vi "JTAG F-RAM Store Trims.vi"(8 "Control F-RAM Power?":bool=TRUE, 9 "Auto-Load this value?":bool=TRUE, 10 "Value to Store":u8 format="%02x", 11 "Trim Location":u16(ring) items=["PWR_TRIM_f0"=0, "PWR_TRIM_1"=1, "PWR_TRIM_2"=2, "PWR_TRIM_3"=3, "PWR_TRIM_4"=4, "PWR_TRIM_5"=5, "PWR_TRIM_6"=6, "PWR_TRIM_7"=7, "PWR_TRIM_8"=8, "PWR_TRIM_9"=9, "PWR_TRIM_10"=10, "STIM_BG_CTRL"=11, "STIM_CG_CTRL"=12, "STIM_PGO_CTRL"=13, "STIM_CM_CTRL"=14, "MICS_TX_RF_POWER"=20, "MICS_TXPORT_TXMODE"=21, "MICS_TXPORT_RXMODE"=22, "MICS_RXPORT_TXMODE"=23, "MICS_RXPORT_RXMODE"=24, "MICS_ANT_MATCH_1"=25, "MICS_ANT_MATCH_2"=26, "MICS_CHANNEL"=27, "MICS_TX_MODULATION"=28, "MICS_MAC_CALSELECT_1"=29, "MICS_MAC_CALSELECT_2"=30]) -> (0 "error out":errorcluster)   [LabVIEW 2009]
panel:
  # "Yes"
  # "No"
  # "Yes"
  # "No"
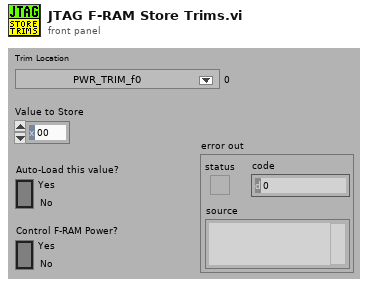
[diagram p1: front panel]
types:
  T1 = enum16{"Power UP", "Power DN", "Read Single", "Write Single", "Read Block", "Write Block", "Read SR", "Write SR", "Send Opcode"}
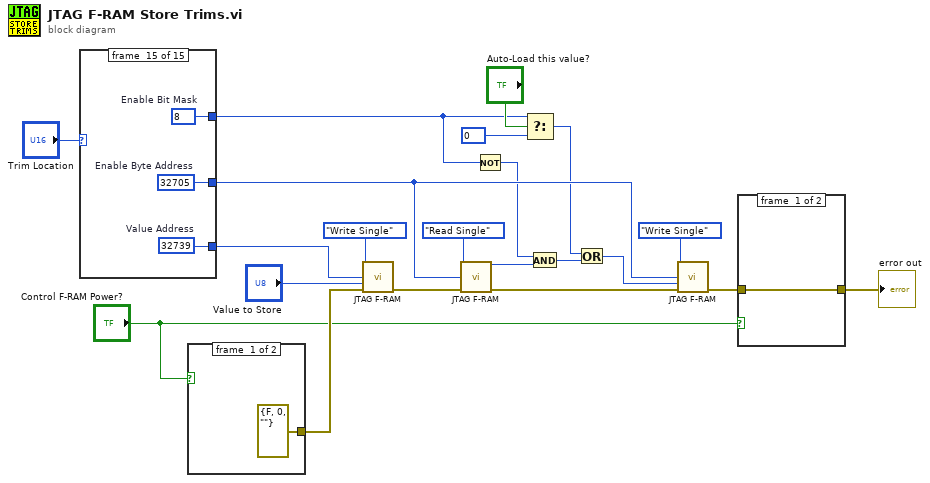
[diagram p0: block diagram]
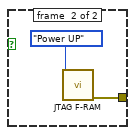
[diagram p2: hidden frame]
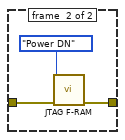
[diagram p3: hidden frame]
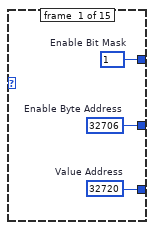
[diagram p4: hidden frame]
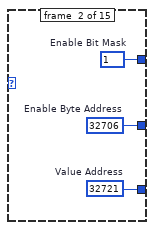
[diagram p5: hidden frame]
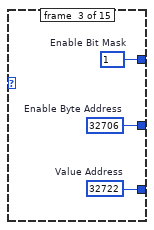
[diagram p6: hidden frame]
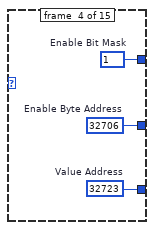
[diagram p7: hidden frame]
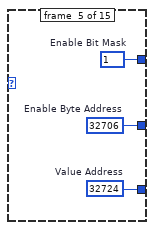
[diagram p8: hidden frame]
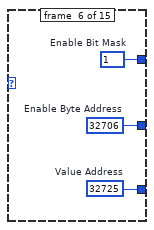
[diagram p9: hidden frame]
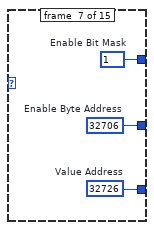
[diagram p10: hidden frame]
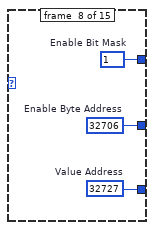
[diagram p11: hidden frame]
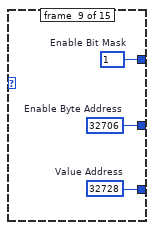
[diagram p12: hidden frame]
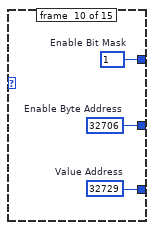
[diagram p13: hidden frame]
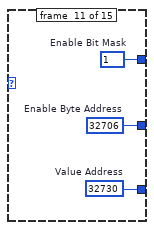
[diagram p14: hidden frame]
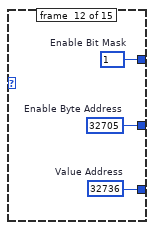
[diagram p15: hidden frame]
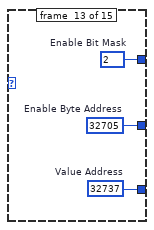
[diagram p16: hidden frame]
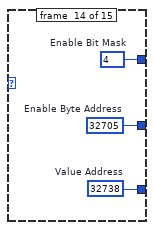
[diagram p17: hidden frame]
diagram:
  n1 = case shown="10" "Trim Location" {
    tunnel: [w24 w27 w30 w33 w36 w39 w42 w45 w48 w51 w54 w57 w60 w63 w66] -> w17
    tunnel: [w23 w26 w29 w32 w35 w38 w41 w44 w47 w50 w53 w56 w59 w62 w65] -> w9
    tunnel: [w22 w25 w28 w31 w34 w37 w40 w43 w46 w49 w52 w55 w58 w61 w64] -> w3
    frame #0 {
      w23 = u16 32706  # Enable Byte Address
      w22 = u8 1  # Enable Bit Mask
      w24 = u16 32720  # Value Address
    }
    frame #1 {
      w26 = u16 32706  # Enable Byte Address
      w25 = u8 1  # Enable Bit Mask
      w27 = u16 32721  # Value Address
    }
    frame #2 {
      w29 = u16 32706  # Enable Byte Address
      w28 = u8 1  # Enable Bit Mask
      w30 = u16 32722  # Value Address
    }
    frame #3 {
      w32 = u16 32706  # Enable Byte Address
      w31 = u8 1  # Enable Bit Mask
      w33 = u16 32723  # Value Address
    }
    frame #4 {
      w35 = u16 32706  # Enable Byte Address
      w34 = u8 1  # Enable Bit Mask
      w36 = u16 32724  # Value Address
    }
    frame #5 {
      w38 = u16 32706  # Enable Byte Address
      w37 = u8 1  # Enable Bit Mask
      w39 = u16 32725  # Value Address
    }
    frame #6 {
      w41 = u16 32706  # Enable Byte Address
      w40 = u8 1  # Enable Bit Mask
      w42 = u16 32726  # Value Address
    }
    frame #7 {
      w44 = u16 32706  # Enable Byte Address
      w43 = u8 1  # Enable Bit Mask
      w45 = u16 32727  # Value Address
    }
    frame #8 {
      w47 = u16 32706  # Enable Byte Address
      w46 = u8 1  # Enable Bit Mask
      w48 = u16 32728  # Value Address
    }
    frame #9 {
      w50 = u16 32706  # Enable Byte Address
      w49 = u8 1  # Enable Bit Mask
      w51 = u16 32729  # Value Address
    }
    frame #10 {
      w53 = u16 32706  # Enable Byte Address
      w52 = u8 1  # Enable Bit Mask
      w54 = u16 32730  # Value Address
    }
    frame #11 {
      w56 = u16 32705  # Enable Byte Address
      w55 = u8 1  # Enable Bit Mask
      w57 = u16 32736  # Value Address
    }
    frame #12 {
      w59 = u16 32705  # Enable Byte Address
      w58 = u8 2  # Enable Bit Mask
      w60 = u16 32737  # Value Address
    }
    frame #13 {
      w62 = u16 32705  # Enable Byte Address
      w61 = u8 4  # Enable Bit Mask
      w63 = u16 32738  # Value Address
    }
    frame #14 {
      w65 = u16 32705  # Enable Byte Address
      w64 = u8 8  # Enable Bit Mask
      w66 = u16 32739  # Value Address
    }
  }
  n2 = case shown="True" "Control F-RAM Power?" {
    tunnel: [errorcluster {"status"=FALSE, "code"=0, "source"=""} ("error out") w68] -> w20
    frame #0 {
    }
    frame #1 {
      n3 = call "JTAG F-RAM.vi"("Function"=T1."Power UP") -> ("error out"=w68:errorcluster)  [unwired: 12 in, 2 out]
    }
  }
  n4 = call "JTAG F-RAM.vi"("Function"=T1."Write Single", "Address"=w17, "Value"="Value to Store", "error in (no error)"=w20) -> ("error out"=w10:errorcluster)  [unwired: 9 in, 2 out]
  n5 = call "JTAG F-RAM.vi"("Function"=T1."Read Single", "Address"=w9, "error in (no error)"=w10) -> ("Read Value"=w6:u8, "error out"=w2:errorcluster)  [unwired: 10 in, 1 out]
  n6 = Not(x=w3) -> (.not. x?=w4:u8)
  n7 = Select(t=w3, s="Auto-Load this value?", f=u8 0) -> (s? t:f=w7:u8)
  n8 = And(x=w4, y=w6) -> (x .and. y?=w5:u8)
  n9 = Or(x=w7, y=w5) -> (x .or. y?=w8:u8)
  n10 = call "JTAG F-RAM.vi"("Function"=T1."Write Single", "Address"=w9, "Value"=w8, "error in (no error)"=w2) -> ("error out"=w13:errorcluster)  [unwired: 9 in, 2 out]
  n11 = case shown="True" "Control F-RAM Power?" {
    tunnel: w13 -> [w70 w72]
    tunnel: [w70 w71] -> w12
    frame #0 {
    }
    frame #1 {
      n12 = call "JTAG F-RAM.vi"("Function"=T1."Power DN", "error in (no error)"=w72) -> ("error out"=w71:errorcluster)  [unwired: 11 in, 2 out]
    }
  }
  "error out" <- w12
